vi "ConditionalEXT.vi"(1 "Value in":ext) -> (0 "Stop?":bool)   [LabVIEW 2017]
doc: "Displays the value of the double-precision, floating-point numeric control and allows conditional breakpoints. If you select multiple conditions, LabVIEW executes a breakpoint if any of those conditions are true."
panel:
  in  "Tab Control":enum32{"Data    ", "Condition     "}(tab)
  out "Value":ext
  in  "Ls":ext
  in  "Gr":ext
  in  "Eq":ext
  in  "Ls":bool
  in  "Gr":bool
  in  "Eq":bool
  # "Pause if any of the following:"
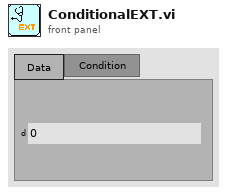
[diagram p1: front panel]
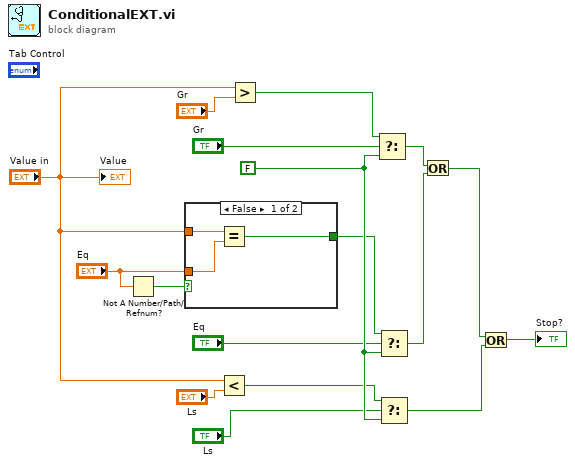
[diagram p0: block diagram]
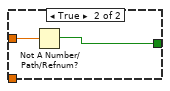
[diagram p2: hidden frame]
diagram:
  w13 = FALSE ("f")
  n1 = Not A Number/Path/Refnum?(number/path/refnum="Eq") -> (NaN/Path/Refnum?=w1:bool)
  n2 = case shown="False" w1 {
    tunnel: [w20 w21] -> w10
    tunnel: "Value in" -> [w19 w22]
    tunnel: "Eq" -> [w18 _]
    frame False {
      n3 = Equal?(x=w19, y=w18) -> (x = y?=w20:bool)
    }
    frame True {
      n4 = Not A Number/Path/Refnum?(number/path/refnum=w22) -> (NaN/Path/Refnum?=w21:bool)
    }
  }
  n5 = Less?(x="Value in", y="Ls") -> (x < y?=w4:bool)
  n6 = Greater?(x="Value in", y="Gr") -> (0:w14:bool)
  n7 = Select(t=w14, s="Gr", f=w13) -> (s? t:f=w8:bool)
  n8 = Select(t=w10, s="Eq", f=w13) -> (s? t:f=w7:bool)
  n9 = Select(t=w4, s="Ls", f=w13) -> (s? t:f=w5:bool)
  n10 = Or(x=w8, y=w7) -> (x .or. y?=w6:bool)
  n11 = Or(x=w6, y=w5) -> (x .or. y?=→"Stop?":bool)
  "Value" <- "Value in"
